vi "VDMS_FPGA_Main_8_Modules_9229.vi"() -> ()   [LabVIEW 2017]
doc: "This VI provides a template for customizing a waveform acquisition using delta-sigma based NI C Series analog input smodules."
uses:
  <vilib>/LabVIEW Targets/FPGA/cRIO/shared/nicrio_ModuleControls/nicrio_cRIO-9232_ConfigModeRing.ctl
  <vilib>/Platform/TimedLoop/XDataNode/timing_clust.ctl
  <vilib>/Platform/TimedLoop/XDataNode/nitl_modes.ctl
  <vilib>/Platform/TimedLoop/XDataNode/wakeup.ctl
  <vilib>/rvi/Emulation/niFpgaGetClockAttributes.vi
  <vilib>/rvi/Emulation/niFpgaSctlEmulationGetInTimedLoop.vi
  <vilib>/rvi/Emulation/niFpgaEmulationReportErrorSimple.vi
  <vilib>/rvi/Emulation/niFpgaProcessEmulError.vi
  <vilib>/addons/InsightCM/Devices/Shared/Cms/Fpga/AcquisitionFpgaTach/source/subVIs/Glbl Stop.vi
  <vilib>/addons/InsightCM/Devices/Shared/Cms/Fpga/AcquisitionFpgaTach/source/subVIs/FPGA Globals.vi
  <vilib>/rvi/eio/common/nirviEmuTemplateMethod_errors.vi
  <vilib>/rvi/Memory/Memory_Emulation/nirvimemoryFastEmulation.vi
  <vilib>/rvi/Memory/Memory_Emulation/nirvimemoryEmulation.vi
  <vilib>/rvi/Emulation/niFpgaEmulationIsFPGAContextNoSignature.vi
  <vilib>/rvi/DataTransferAndStorage/Container/Common/niFpgaContainerGetUniqueNameForEmu.vi
  <vilib>/rvi/errors/nirviReportUnexpectedCaseInternalError (U32).vi
  <vilib>/rvi/DataTransferAndStorage/Container/Common/niFpgaContainerExecOnDevCompGetState.vi
  <vilib>/rvi/Memory/Memory_Emulation/niFpgaMemoryEmulationCacheClearOnFirstRun.vi
  <vilib>/rvi/Memory/Memory_Emulation/nirvimemoryEmulationManagerCache_MakeExclusive.vi
  <vilib>/rvi/Memory/Memory_Emulation/niFpgaMemoryEmulationValidateCache.vi
  <vilib>/rvi/Memory/Memory_Emulation/nirvimemoryEmulationManagerCache_InsertValue.vi
  <vilib>/Utility/error.llb/Clear Errors.vi
  <vilib>/rvi/Memory/Memory_Emulation/nirvimemoryEmulationManagerCache_ReleaseExclusive.vi
  <vilib>/rvi/Memory/Memory_Emulation/nirvimemoryEmulationManagerCache_GetValue.vi
  <vilib>/rvi/Memory/Memory_Emulation/nirvimemoryEmulationManagerCache_SetValue.vi
  <vilib>/rvi/Emulation/niFpgaSctlEmulationResourceMgr.vi
  <vilib>/rvi/Emulation/niFpgaCriticalErrorInLSC.vi
  <vilib>/rvi/interface/RandomDataEmulation/niFpgaRandomDataHandleErrors.vi
  <vilib>/rvi/errors/niFpgaSetErrorForExecOnDevCompSimple.vi
  <vilib>/rvi/eio/common/nirviEmuReportErrorAndStop.vi
  <vilib>/rvi/FIFO/Fifo_Resource/nirvififoEmulationSetSize.vi
  <vilib>/rvi/FIFO/Fifo_Resource/nirviFifoEmulationQueueMgr.vi
  <instcachedir>/0/nirviFifoEmulationQueueMgr_E5CAEC123FF24DC58D834DCA3CDAA9B5.lvgen/nirviFifoEmulationQueueMgr_E5CAEC123FF24DC58D834DCA3CDAA9B5_001.vi
  <vilib>/rvi/FIFO/Fifo_Resource/nirvififoEmulationDetermineInputValidOut.vi
  <vilib>/rvi/FIFO/Fifo_Resource/nirvififoEmulationCreateLock.vi
  <vilib>/rvi/FIFO/Fifo_Resource/nirvififoEmulationObtainLock.vi
  <vilib>/rvi/FIFO/Fifo_Resource/nirvififoEmulationReleaseLock.vi
  <vilib>/rvi/occurrence/nirviWaitOnOccurrenceBase.vi
  <vilib>/rvi/errors/nirviReportUnexpectedCaseInternalError.vi
  <vilib>/eio/EIONode/EIONode.xnode
  <vilib>/rvi/DataTransferAndStorage/Container/XNode/niFpgaContainer.xnode
  <vilib>/rvi/Memory/Memory_Emulation/niFpgaMemoryEmulationRefIn.vi
  <vilib>/Platform/TimedLoop/XDataNode/XDataNode.xnode
  <vilib>/rvi/interface/RandomDataEmulation/nirviRandomDataFpgaReadWriteTemplate.vi
  <vilib>/rvi/FXPMathLib/basic elements/FxpDiscreteDelay/XNode/nifxpmath_DiscreteDelay.xnode
  <vilib>/rvi/FIFO/Fifo_Resource/niFpgaFifoEmulationRefIn.vi
  <vilib>/Platform/TimedLoop/XDataNode/XDNodeRunTimeDep.lvlib
  <vilib>/addons/InsightCM/Devices/Shared/Cms/Fpga/AcquisitionFpgaTach/source/subVIs/VibAPI_8/VDMS_VibAPI_8.lvlib
panel:
  in  "Tach Delay":u8
  out "Chassis Temperature":sgl
  in  "Enable Chan Array":bool[](array[boolean])=[FALSE, FALSE, FALSE, FALSE, FALSE, FALSE, FALSE, FALSE, FALSE, FALSE, FALSE, FALSE, FALSE, FALSE, FALSE, FALSE, FALSE, FALSE, FALSE, FALSE, FALSE, FALSE, FALSE, FALSE, FALSE, FALSE, FALSE, FALSE, FALSE, FALSE, FALSE, FALSE]
  in  "Custom Scale Intercept":sgl[](array[numeric])=[0.0, 0.0, 0.0, 0.0, 0.0, 0.0, 0.0, 0.0, 0.0, 0.0, 0.0, 0.0, 0.0, 0.0, 0.0, 0.0, 0.0, 0.0, 0.0, 0.0, 0.0, 0.0, 0.0, 0.0, 0.0, 0.0, 0.0, 0.0, 0.0, 0.0, 0.0, 0.0]
  in  "Custom Scale Slope":sgl[](array[numeric])=[0.0, 0.0, 0.0, 0.0, 0.0, 0.0, 0.0, 0.0, 0.0, 0.0, 0.0, 0.0, 0.0, 0.0, 0.0, 0.0, 0.0, 0.0, 0.0, 0.0, 0.0, 0.0, 0.0, 0.0, 0.0, 0.0, 0.0, 0.0, 0.0, 0.0, 0.0, 0.0]
  in  "Threshold2":fxp<+/-,24,7>=-10.0
  in  "Slope2":enum16{"falling", "rising"}(ring)
  in  "Hysteresis2":fxp<+/-,24,7>=1.0
  in  "Hysteresis1":fxp<+/-,24,7>=1.0
  in  "Threshold1":fxp<+/-,24,7>=-10.0
  in  "Slope1":enum16{"falling", "rising"}(ring)
  in  "Hysteresis0":fxp<+/-,24,7>=1.0
  in  "Slope0":enum16{"falling", "rising"}(ring)
  in  "Threshold0":fxp<+/-,24,7>=-10.0
  out "Tach FIFO Full":bool
  in  "Delay Comp":u32
  out "Start Trigger":bool
  in  "Number of Modules":i16=1
  out "Open Loop Chan Array":bool[](array[boolean])
  out "Short Circuit Chan Array":bool[](array[boolean])
  in  "Input Config Array":T1[](array[typedef])=[1, 1, 1, 1, 1, 1, 1, 1, 1, 1, 1, 1, 1, 1, 1, 1, 1, 1, 1, 1, 1, 1, 1, 1, 0, 0, 0, 0, 0, 0, 0, 0] items=["AC Coupled", "DC Coupled", "IEPE AC Coupled"]
  in  "Data Rate [S/s]":u32=1280
  out "Chan Count":bool
  out "Acq Loop Ticks":u32
  out "FPGA Error":errorcluster
  out "Module Underflow":bool
  out "Finished":bool
  in  "Total Avail Channels":i32=4
  in  "Samps per Chan [Finite]":i32=5120
  out "First Read":bool
  in  "Acquisition Type":enum16{"Finite Samples", "Continuous Samples"}(ring)
  out "DMA FIFO Full":bool
  in  "Stop":bool
  # "Keyphasor Info"
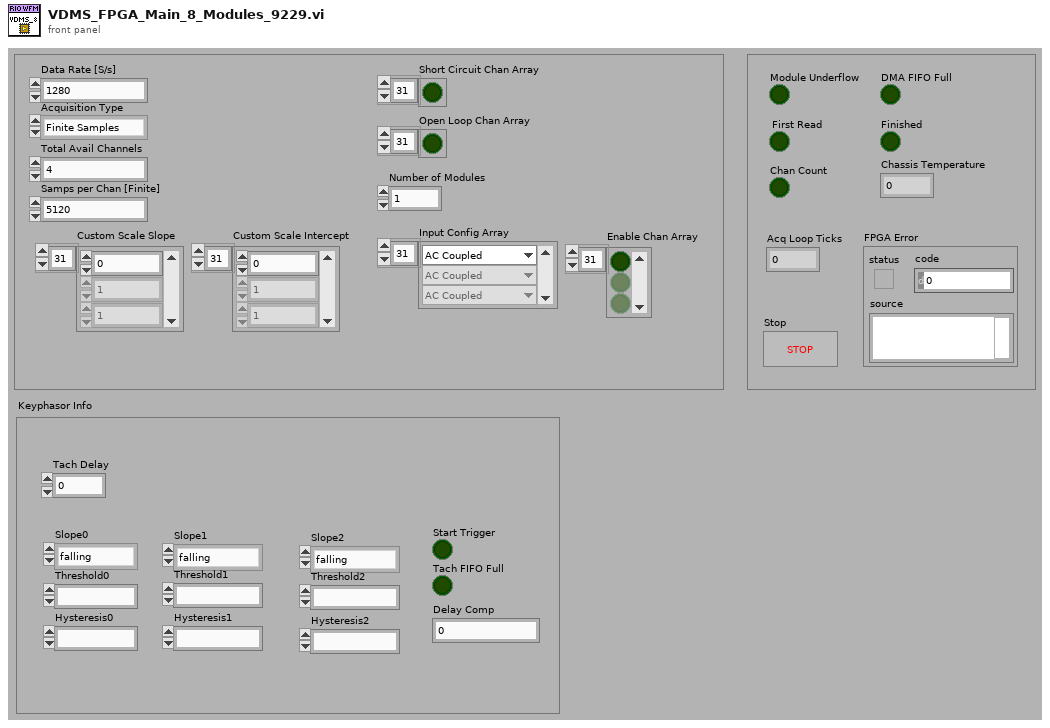
[diagram p1: front panel]
types:
  T1 = typedef "nicrio_cRIO-9232_ConfigModeRing.ctl" = u8
  T2 = typedef "XDNodeRunTimeDep.lvlib/timing_clust.ctl" = cluster{"Expected End [f-1]":u64, "Actual End [f-1]":u64, "Finished Late? [f-1]":bool, "Expected End [i-1]":u64, "Actual End [i-1]":u64, "Finished Late? [i-1]":bool, "Expected Start [i]":u64, "Actual Start [i]":u64, "Expected Start [f]":u64, "Actual Start [f]":u64, "Source Name":string, "Structure Name":string, "Period":i64, "Deadline":i64, "Offset":i64, "Start":i64, "Priority":i32, "Timeout":i32, "Mode":T3, "Wakeup Reason":T4, "Error":errorcluster, "Source Type":string, "Secondary Source Type":string, "Global End Time":u64, "Global Start Time":u64, "Frame Duration":u64, "Iteration Duration":u64, "Assigned CPU":i32, "I/O Scan Engine Mode":u32}
  T3 = typedef "XDNodeRunTimeDep.lvlib/nitl_modes.ctl" = enum32{"No Change", "Process missed periods, maintain original phase", "Discard missed periods, maintain original phase", "Process missed periods, ignore original phase", "Discard missed periods, ignore original phase"}
  T4 = typedef "XDNodeRunTimeDep.lvlib/wakeup.ctl" = enum32{"Normal", "Aborted", "Asynchronous wakeup", "Timing source error", "Timed loop error", "Timeout"}
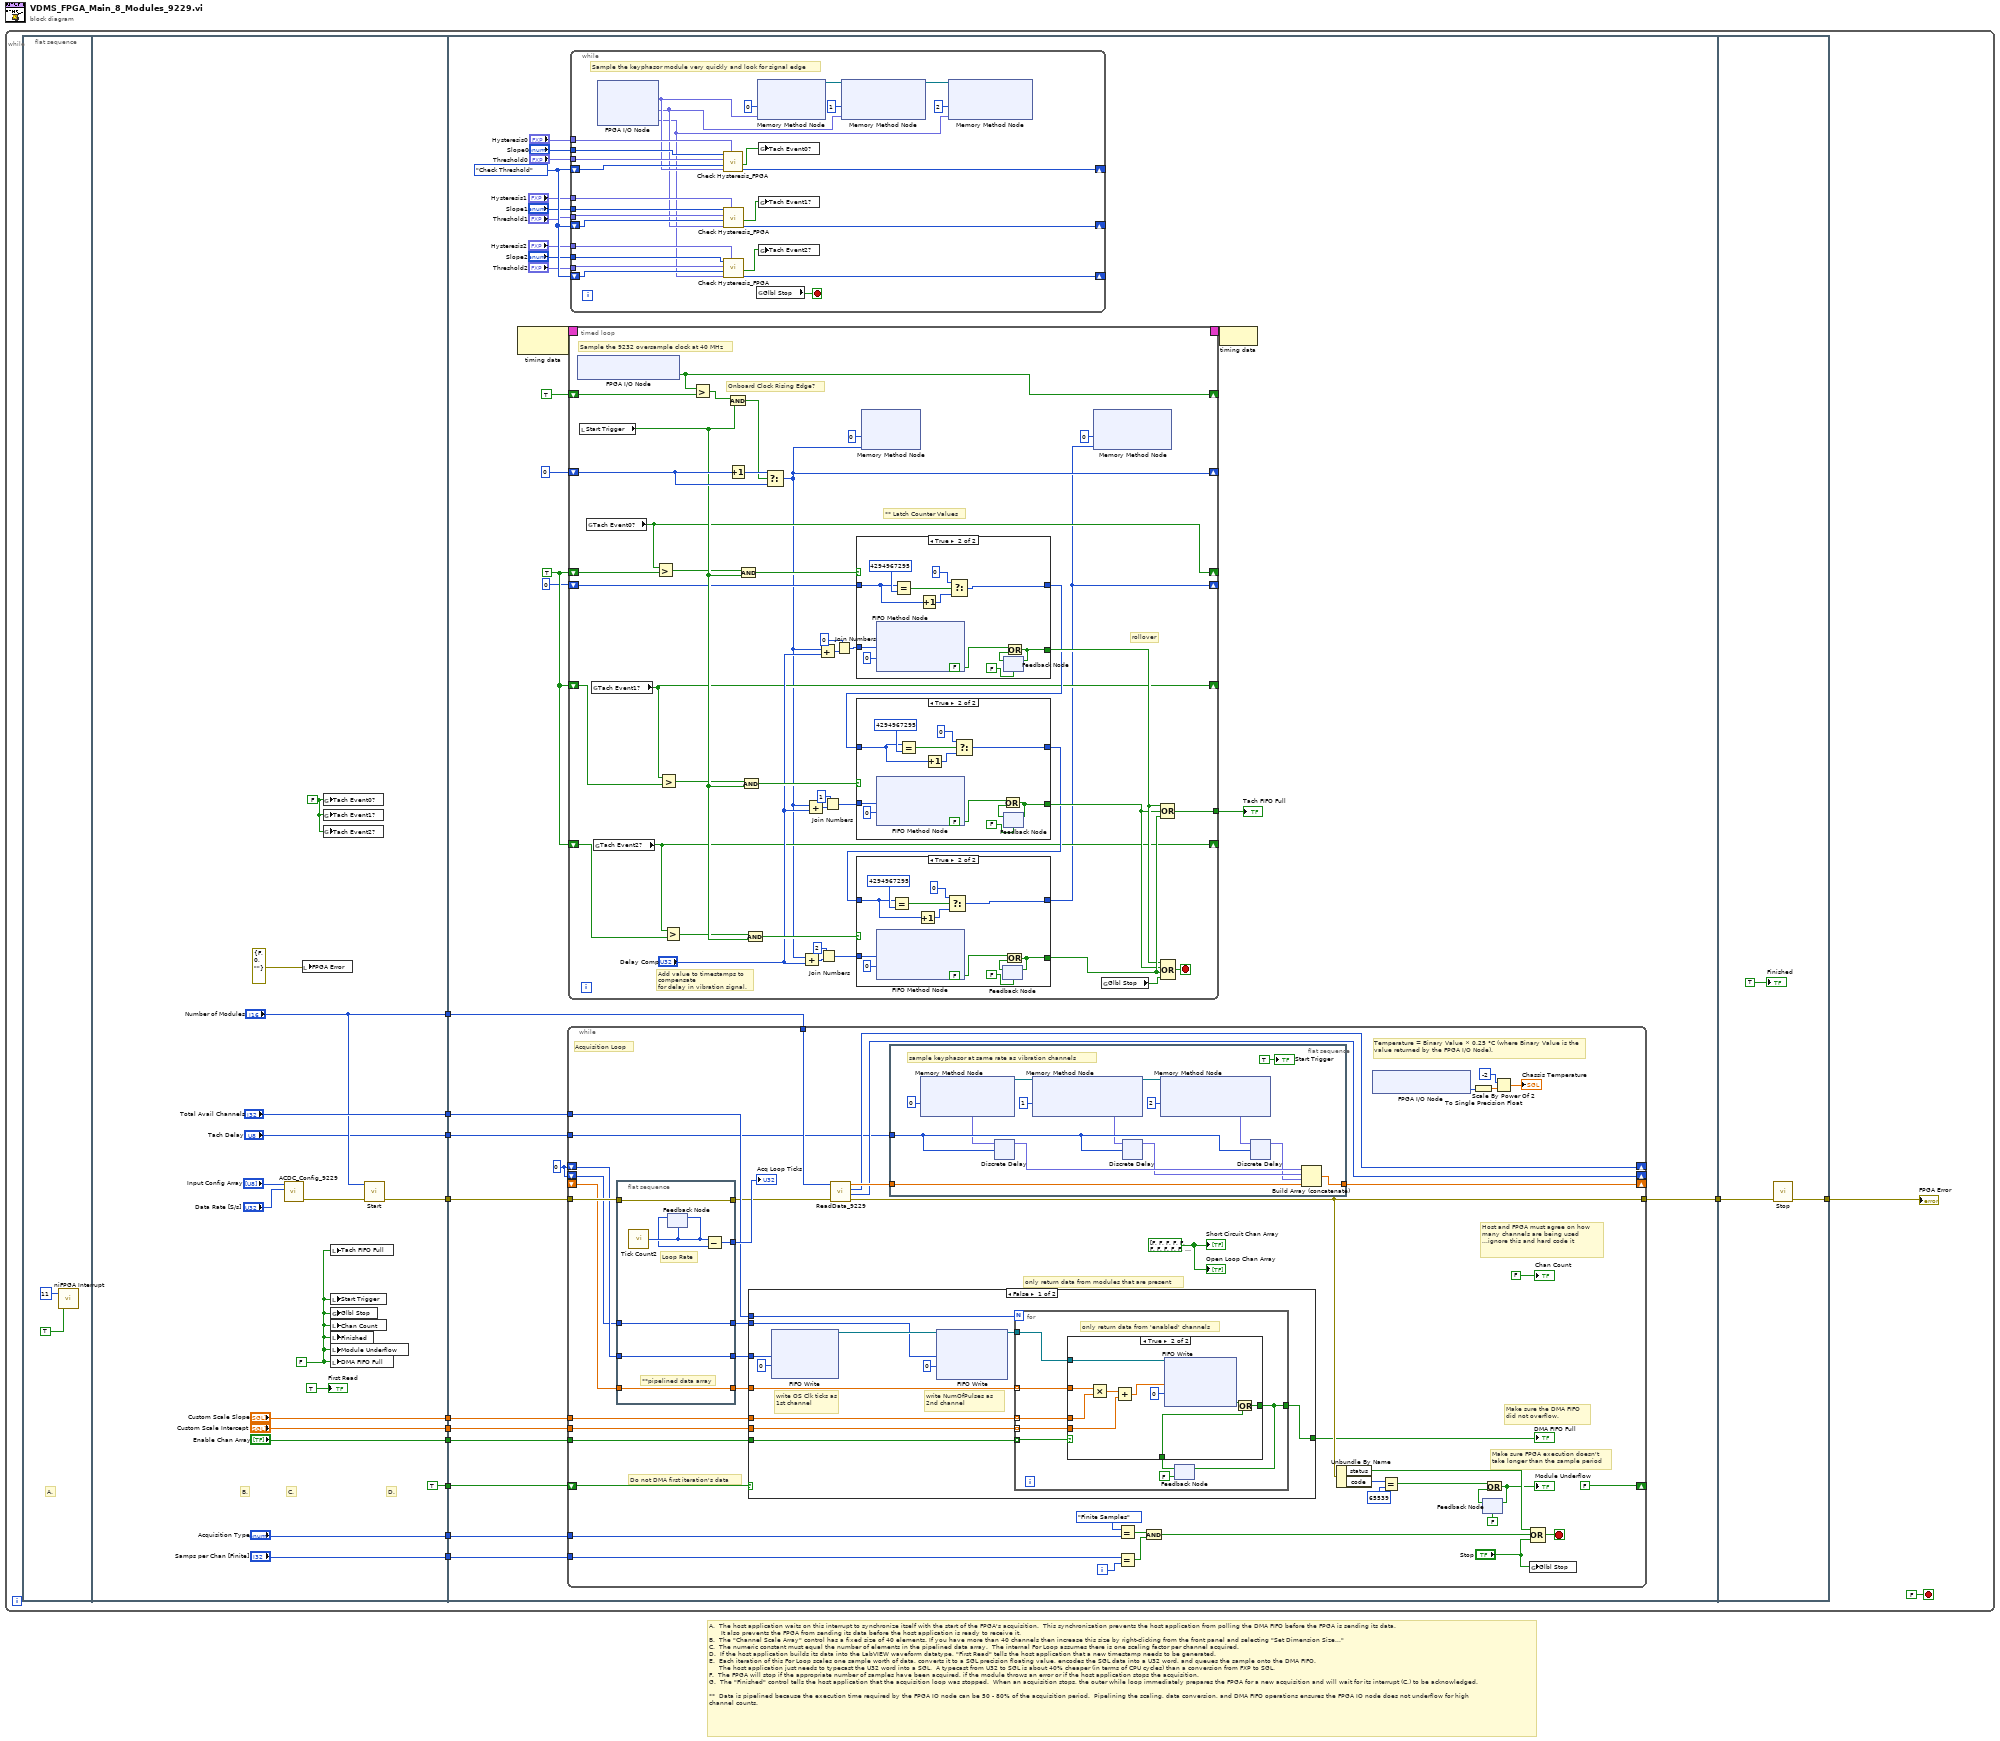
[diagram p0: block diagram]
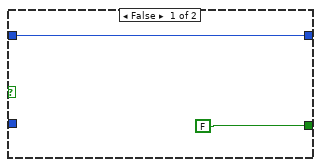
[diagram p2: hidden frame]
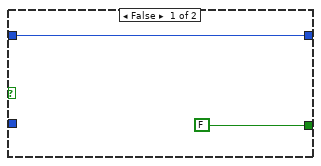
[diagram p3: hidden frame]
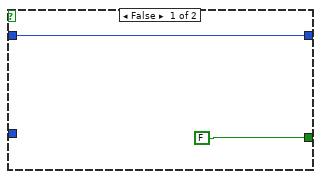
[diagram p4: hidden frame]
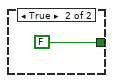
[diagram p6: hidden frame]
diagram:
  # "A.  The host application waits on this interrupt to synchronize itself with the start of the FPGA's acquisition.  This synchronization prevents the host application from polling the DMA FIFO before the FPGA is sending its data.\n      It also prevents the FPGA from sending its data before the host application is ready to receive it.\nB.  The \"Channel Scale Array\" control has a fixed size of 40 elements. If you have more than 40 channels then increase this size by right-clicking from the front panel and selecting \"Set Dimension Size...\"\nC.  The numeric constant must equal the number of elements in the pipelined data array.  The internal For Loop assumes there is one scaling factor per channel acquired.  \nD.  If the host application builds its data into the LabVIEW waveform datatype, \"First Read\" tells the host application that a new timestamp needs to be generated.\nE.  Each iteration of this For Loop scales one sample worth of data, converts it to a SGL precision floating value, encodes the SGL data into a U32 word, and queues the sample onto the DMA FIFO.  \n     The host application just needs to typecast the U32 word into a SGL.  A typecast from U32 to SGL is about 40% cheaper (in terms of CPU cycles) than a conversion from FXP to SGL.\nF.  The FPGA will stop if the appropriate number of samples have been acquired, if the module throws an error or if the host application stops the acquisition.  \nG.  The \"Finished\" control tells the host application that the acquisition loop was stopped.  When an acquisition stops, the outer while loop immediately prepares the FPGA for a new acquisition and will wait for its interrupt (C.) to be acknowledged.\n\n**  Data is pipelined because the execution time required by the FPGA IO node can be 50 - 80% of the acquisition period.  Pipelining the scaling, data conversion, and DMA FIFO operations ensures the FPGA IO node does not underflow for high\nchannel counts."
  n1 = while {
    stop <- FALSE stop-if-true
    n2 = flat-sequence {
      tunnel: [w26] -> w12
      tunnel: ["Acquisition Type"] -> w11
      tunnel: ["Samps per Chan [Finite]"] -> w10
      tunnel: ["Total Avail Channels"] -> w9
      tunnel: [TRUE ("t")] -> w8
      tunnel: ["Number of Modules"] -> w6
      tunnel: ["Custom Scale Slope"] -> w4
      tunnel: ["Custom Scale Intercept"] -> w3
      tunnel: ["Enable Chan Array"] -> w2
      tunnel: ["Tach Delay"] -> w1
      tunnel: w12 -> [w60]
      tunnel: w11 -> [w58]
      tunnel: w10 -> [w57]
      tunnel: w9 -> [w61]
      tunnel: w8 -> [w59]
      tunnel: [w56] -> w7
      tunnel: w6 -> [w55]
      tunnel: w4 -> [w38]
      tunnel: w3 -> [w37]
      tunnel: w2 -> [w36]
      tunnel: w1 -> [w33]
      tunnel: w7 -> [w277]
      tunnel: [w276] -> w5
      frame #0 {
        # "A."
        n3 = call <vilib>:"niFPGA Interrupt.vi"("Wait Until Cleared (F)"=TRUE ("Wait Until Cleared"), "IRQ Number (0)"=u8 11 ("IRQ Number")) -> ()  [unwired: 1 in]
      }
      frame #1 {
        w17 = FALSE ("Tach Event0?")
        w22 = FALSE ("Module Underflow")
        # "D."
        # "C."
        # "B."
        n4 = call <vilib>:"ACDC_Config_9229.vi"("Data Rate [S/s]"="Data Rate [S/s]", "Input Config Array"="Input Config Array") -> ("error out"=w25:errorcluster)  [unwired: 9 in]
        n5 = local write "FPGA Error"(errorcluster {"status"=FALSE, "code"=0, "source"=""} ("FPGA Error")) -> ()
        n6 = global write "FPGA Globals.vi" "Tach Event0?"(w17) -> ()
        n7 = global write "FPGA Globals.vi" "Tach Event1?"(w17) -> ()
        n8 = global write "FPGA Globals.vi" "Tach Event2?"(w17) -> ()
        n9 = local write "Tach FIFO Full"(w22) -> ()
        n10 = local write "Start Trigger"(w22) -> ()
        n11 = global write "Glbl Stop.vi" "Glbl Stop"(w22) -> ()
        n12 = local write "Chan Count"(w22) -> ()
        n13 = local write "Finished"(w22) -> ()
        n14 = local write "Module Underflow"(w22) -> ()
        n15 = local write "DMA FIFO Full"(w22) -> ()
        n16 = call <vilib>:"Start.vi"("error in (no error)"=w25, "Module Config Selector"="Number of Modules") -> ("error out"=w26:errorcluster)  [unwired: 9 in]
        "First Read" <- TRUE ("First Read")
      }
      frame #2 {
        w34 = u32 0 ("OversampleClk Ticks")
        w46 = enum16{"Check Hysteresis", "Check Threshold"}."Check Threshold" ("State Out")
        w50 = TRUE
        n17 = node-c288() -> (w54:T2)  [unwired: 1 out]
        n18 = while {
          tunnel: w60 -> [w213]
          tunnel: [w215] -> w56
          tunnel: w58 -> [w217]
          tunnel: w57 -> [w216]
          shift-right: [w192] -> _
          shift-left: _ -> [w210]
          tunnel: w61 -> [w196]
          shift-right: [FALSE ("t")] -> _
          shift-left: w59 -> [w209]
          tunnel: w55 -> [w197]
          shift-right: [w191] -> _
          shift-left: w34 -> [w190]
          tunnel: w38 -> [w188]
          tunnel: w37 -> [w187]
          tunnel: w36 -> [w186]
          shift-right: [w185] -> _
          shift-left: w34 -> [w184]
          tunnel: w33 -> [w178]
          i -> [w207]
          stop <- w220 stop-if-true
          w177 = bool[] [FALSE, FALSE, FALSE, FALSE, FALSE, FALSE, FALSE, FALSE, FALSE, FALSE, FALSE, FALSE, FALSE, FALSE, FALSE, FALSE, FALSE, FALSE, FALSE, FALSE, FALSE, FALSE, FALSE, FALSE, FALSE, FALSE, FALSE, FALSE, FALSE, FALSE, FALSE, FALSE] ("Short Circuit Chan Array")
          # "Temperature = Binary Value × 0.25 °C (where Binary Value is the value returned by the FPGA I/O Node)."
          # "only return data from modules that are present"
          # "Do not DMA first iteration's data"
          # "Acquisition Loop"
          # "Host and FPGA must agree on how \nmany channels are being used\n...ignore this and hard code it"
          # "Make sure the DMA FIFO\ndid not overflow."
          # "Make sure FPGA execution doesn't\ntake longer than the sample period"
          n19 = flat-sequence {
            tunnel: w213 -> [w271]
            tunnel: [w273] -> w212
            tunnel: w210 -> [w272]
            tunnel: [w272] -> w211
            tunnel: [w271] -> w194
            tunnel: [w270] -> w189
            tunnel: w190 -> [w270]
            tunnel: [w269] -> w183
            tunnel: w184 -> [w269]
            frame #0 {
              # "**pipelined data array"
              # "Loop Rate"
              n20 = call "Tick Count2"() -> ("Tick Count(Ticks)"=w275:u32)
              n21 = feedback-in #1(w275) -> ()
              n22 = feedback #1(w275) -> (w274:u32)
              n23 = Subtract(x=w275, y=w274) -> (x-y=w273:u32)
            }
          }
          n24 = case shown="False" w209 {
            tunnel: [w241 FALSE] -> w214
            tunnel: w211 -> [w245 _]
            tunnel: w196 -> [w246 _]
            tunnel: w189 -> [w247 _]
            tunnel: w188 -> [w244 _]
            tunnel: w187 -> [w243 _]
            tunnel: w186 -> [w242 _]
            tunnel: w183 -> [w237 _]
            frame False {
              # "write NumOfPulses as 2nd channel"
              # "write OS Clk ticks as 1st channel"
              n25 = xnode ("FIFO Write")("Element"=w247, "Timeout"=0) -> ("FIFO Out"=w240:refnum<k21>)  [unwired: 1 in, 1 out]
              n26 = xnode ("FIFO Write")("Element"=w237, "Timeout"=0, "FIFO In"=w240) -> ("FIFO Out"=w238:refnum<k21>)  [unwired: 1 out]
              n27 = for {
                N: w246 -> [_]
                tunnel: [w255] -> w241
                tunnel: w245 -> [w254] mode=indexing
                tunnel: w244 -> [w253] mode=indexing
                tunnel: w242 -> [w251] mode=indexing
                tunnel: w243 -> [w250] mode=indexing
                tunnel: w238 -> [w249]
                # "only return data from 'enabled' channels"
                n28 = feedback #2(FALSE) -> (w256:bool)
                n29 = case shown="True" w251 {
                  tunnel: w256 -> [w257 w267]
                  tunnel: [w257 w266] -> w255
                  tunnel: w254 -> [_ w265]
                  tunnel: w253 -> [_ w264]
                  tunnel: w250 -> [_ w259]
                  tunnel: w249 -> [_ w258]
                  frame False {
                  }
                  frame True {
                    n30 = Multiply(x=w265, y=w264) -> (x*y=w261:sgl)
                    n31 = Add(x=w261, y=w259) -> (x+y=w260:sgl)
                    n32 = xnode ("FIFO Write")("Element"=w260, "Timeout"=0, "FIFO In"=w258) -> ("Timed Out?"=w262:bool)  [unwired: 1 out]
                    n33 = Or(x=w262, y=w267) -> (x .or. y?=w266:bool)
                  }
                }
                n34 = feedback-in #2(w255) -> ()
              }
            }
            frame True {
            }
          }
          "DMA FIFO Full" <- w214
          n35 = call <vilib>:"ReadData_9229.vi"("error in"=w194, "Module Config Selector"=w197) -> ("error out"=w215:errorcluster, "Number Of Pulses"=w185:u32, "OversampleClk Ticks"=w191:u32, "Data Array"=w193:sgl[])  [unwired: 6 in]
          n36 = flat-sequence {
            tunnel: w193 -> [w236]
            tunnel: [w235] -> w192
            tunnel: w178 -> [w228]
            frame #0 {
              # "sample keyphasor at same rate as vibration channels"
              n37 = xnode ("Memory Method Node")("Address"=u32 0) -> ("Data"=w227:fxp<+/-,24,7>, "Memory Out"=w232:refnum<k21>)  [unwired: 1 in]
              n38 = xnode ("Discrete Delay")("D"=w227, "n-1[0..41]"=w228) -> ("Q"=w226:fxp<+/-,24,7>)
              n39 = xnode ("Memory Method Node")("Address"=u32 1, "Memory In"=w232) -> ("Data"=w225:fxp<+/-,24,7>, "Memory Out"=w231:refnum<k21>)
              n40 = xnode ("Discrete Delay")("D"=w225, "n-1[0..41]"=w228) -> ("Q"=w224:fxp<+/-,24,7>)
              n41 = xnode ("Memory Method Node")("Address"=u32 2, "Memory In"=w231) -> ("Data"=w223:fxp<+/-,24,7>)  [unwired: 1 out]
              n42 = xnode ("Discrete Delay")("D"=w223, "n-1[0..41]"=w228) -> ("Q"=w222:fxp<+/-,24,7>)
              n43 = Build Array (concatenate)(w226, w224, w222, w236) -> (w235:sgl[])
              "Start Trigger" <- TRUE ("Start Trigger")
            }
          }
          n44 = Equal?(x=enum16{"Finite Samples", "Continuous Samples"}."Finite Samples" ("y"), y=w217) -> (x = y?=w201:bool)
          n45 = Equal?(x=w216, y=w207) -> (x = y?=w200:bool)
          n46 = And(x=w201, y=w200) -> (x .and. y?=w199:bool)
          n47 = Unbundle By Name(w215) -> ("status"=w206:bool, "code"=w218:i32)
          n48 = xnode "FPGA I/O Node"() -> ("Chassis Temperature"=w180:i16)  [unwired: 1 in, 1 out]
          n49 = Equal?(x=w218, y=65539) -> (x = y?=w203:bool)
          n50 = To Single Precision Float(number=w180) -> (single precision float=w182:sgl)
          n51 = feedback #3(FALSE) -> (w205:bool)
          n52 = Or(x=w203, y=w205) -> (x .or. y?=w202:bool)
          "Module Underflow" <- w202
          n53 = feedback-in #3(w202) -> ()
          n54 = Scale By Power Of 2(n=i16 -2, x=w182) -> (x*2^n=→"Chassis Temperature":sgl)
          n55 = global write "Glbl Stop.vi" "Glbl Stop"("Stop") -> ()
          n56 = Compound Arithmetic op=OR(w206, w199, "Stop") -> (w220:bool)
          "Chan Count" <- FALSE ("Chan Count")
          "Acq Loop Ticks" <- w212
          "Short Circuit Chan Array" <- w177
          "Open Loop Chan Array" <- w177
        }
        n57 = timed-loop {
          timing: w54 -> [_]
          timing-out: [_] -> w53
          shift-right: [w92] -> _
          shift-left: u32 0 -> [w127]
          shift-right: [w129] -> _
          shift-left: TRUE -> [w130]
          shift-right: [w95] -> _
          shift-left: w50 -> [w126]
          shift-right: [w94] -> _
          shift-left: w50 -> [w120]
          shift-right: [w93] -> _
          shift-left: w50 -> [w119]
          tunnel: [w101] -> w39
          shift-right: [w91] -> _
          shift-left: u32 0 -> [w98]
          stop <- w125 stop-if-true
          # "rollover"
          # "** Latch Counter Values"
          # "Add value to timestamps to compensate \nfor delay in vibration signal."
          # "Sample the 9232 oversample clock at 40 MHz"
          # "Onboard Clock Rising Edge?"
          n58 = xnode "FPGA I/O Node"() -> ("Mod1/Onboard Clock"=w129:bool)  [unwired: 1 in, 1 out]
          n59 = local read "Start Trigger"() -> (w118:bool)
          n60 = global read "FPGA Globals.vi" "Tach Event0?"() -> (w95:bool)
          n61 = global read "FPGA Globals.vi" "Tach Event1?"() -> (w94:bool)
          n62 = global read "FPGA Globals.vi" "Tach Event2?"() -> (w93:bool)
          n63 = Greater?(x=w95, y=w126) -> (0:w117:bool)
          n64 = Greater?(x=w94, y=w120) -> (0:w116:bool)
          n65 = Greater?(x=w93, y=w119) -> (0:w115:bool)
          n66 = Greater?(x=w129, y=w130) -> (0:w124:bool)
          n67 = And(x=w124, y=w118) -> (x .and. y?=w123:bool)
          n68 = Increment(x=w127) -> (x+1=w128:u32)
          n69 = And(x=w117, y=w118) -> (x .and. y?=w114:bool)
          n70 = And(x=w116, y=w118) -> (x .and. y?=w112:bool)
          n71 = And(x=w115, y=w118) -> (x .and. y?=w106:bool)
          n72 = Select(t=w128, s=w123, f=w127) -> (s? t:f=w92:u32)
          n73 = Add(x=w92, y="Delay Comp") -> (x+y=w108:u32)
          n74 = Add(x=w92, y="Delay Comp") -> (x+y=w111:u32)
          n75 = Add(x=w92, y="Delay Comp") -> (x+y=w122:u32)
          n76 = Join Numbers(hi=u32 2, lo=w108) -> ((hi.lo)=w104:u64)
          n77 = Join Numbers(hi=u32 1, lo=w111) -> ((hi.lo)=w109:u64)
          n78 = Join Numbers(hi=u32 0, lo=w122) -> ((hi.lo)=w121:u64)
          n79 = case shown="True" w114 {
            tunnel: [FALSE w171] -> w100
            tunnel: w121 -> [_ w168]
            tunnel: w98 -> [w159 w164]
            tunnel: [w159 w161] -> w97
            frame False {
            }
            frame True {
              (unwired) FALSE
              n80 = xnode ("FIFO Method Node")("Element"=w168, "Timeout"=0) -> ("Timed Out?"=w169:bool)  [unwired: 1 in, 1 out]
              n81 = Equal?(x=w164, y=u32 4294967295) -> (x = y?=w165:bool)
              n82 = Increment(x=w164) -> (x+1=w163:u32)
              n83 = Select(t=u32 0, s=w165, f=w163) -> (s? t:f=w161:u32)
              n84 = feedback #4(FALSE) -> (w172:bool)
              n85 = Or(x=w169, y=w172) -> (x .or. y?=w171:bool)
              n86 = feedback-in #4(w171) -> ()
            }
          }
          n87 = case shown="True" w112 {
            tunnel: [FALSE w157] -> w99
            tunnel: w109 -> [_ w154]
            tunnel: w97 -> [w145 w148]
            tunnel: [w145 w147] -> w96
            frame False {
            }
            frame True {
              (unwired) FALSE
              n88 = xnode ("FIFO Method Node")("Element"=w154, "Timeout"=0) -> ("Timed Out?"=w155:bool)  [unwired: 1 in, 1 out]
              n89 = Equal?(x=w148, y=u32 4294967295) -> (x = y?=w150:bool)
              n90 = Increment(x=w148) -> (x+1=w151:u32)
              n91 = Select(t=u32 0, s=w150, f=w151) -> (s? t:f=w147:u32)
              n92 = feedback #5(FALSE) -> (w158:bool)
              n93 = Or(x=w155, y=w158) -> (x .or. y?=w157:bool)
              n94 = feedback-in #5(w157) -> ()
            }
          }
          n95 = case shown="True" w106 {
            tunnel: [FALSE w143] -> w102
            tunnel: w104 -> [_ w140]
            tunnel: w96 -> [w131 w134]
            tunnel: [w131 w133] -> w91
            frame False {
            }
            frame True {
              (unwired) FALSE
              n96 = xnode ("FIFO Method Node")("Element"=w140, "Timeout"=0) -> ("Timed Out?"=w141:bool)  [unwired: 1 in, 1 out]
              n97 = Equal?(x=w134, y=u32 4294967295) -> (x = y?=w137:bool)
              n98 = Increment(x=w134) -> (x+1=w136:u32)
              n99 = Select(t=u32 0, s=w137, f=w136) -> (s? t:f=w133:u32)
              n100 = feedback #6(FALSE) -> (w144:bool)
              n101 = Or(x=w141, y=w144) -> (x .or. y?=w143:bool)
              n102 = feedback-in #6(w143) -> ()
            }
          }
          n103 = xnode ("Memory Method Node")("Address"=u32 0, "Data"=w92) -> ()  [unwired: 1 in, 1 out]
          n104 = xnode ("Memory Method Node")("Address"=u32 0, "Data"=w91) -> ()  [unwired: 1 in, 1 out]
          n105 = global read "Glbl Stop.vi" "Glbl Stop"() -> (w103:bool)
          n106 = Compound Arithmetic op=OR(w100, w99, w102) -> (w101:bool)
          n107 = Compound Arithmetic op=OR(w100, w99, w102, w103) -> (w125:bool)
        }
        "Tach FIFO Full" <- w39
        n108 = while {
          shift-right: [w86] -> _
          shift-left: w46 -> [w87]
          tunnel: "Slope0" -> [w85]
          tunnel: "Threshold0" -> [w84]
          tunnel: "Hysteresis0" -> [w83]
          shift-right: [w82] -> _
          shift-left: w46 -> [w80]
          shift-right: [w81] -> _
          shift-left: w46 -> [w79]
          tunnel: "Hysteresis1" -> [w78]
          tunnel: "Slope1" -> [w77]
          tunnel: "Threshold1" -> [w76]
          tunnel: "Hysteresis2" -> [w75]
          tunnel: "Slope2" -> [w74]
          tunnel: "Threshold2" -> [w73]
          stop <- w88 stop-if-true
          # "Sample the keyphasor module very quickly and look for signal edge"
          n109 = xnode "FPGA I/O Node"() -> ("Mod1/AI0"=w64:fxp<+/-,24,7>, "Mod1/AI1"=w63:fxp<+/-,24,7>, "Mod1/AI2"=w62:fxp<+/-,24,7>)  [unwired: 3 in, 3 out]
          n110 = call <vilib>:"Check Hysteresis_FPGA.vi"("Hysteresis"=w83, "Analog In (Tach)"=w64, "State In"=w87, "Threshold"=w84, "Slope"=w85) -> ("State Out"=w86:enum16{"Check Hysteresis", "Check Threshold"}, "Event Ocurred?"=w71:bool)  [unwired: 2 in]
          n111 = call <vilib>:"Check Hysteresis_FPGA.vi"("Hysteresis"=w78, "Analog In (Tach)"=w63, "State In"=w80, "Threshold"=w76, "Slope"=w77) -> ("State Out"=w82:enum16{"Check Hysteresis", "Check Threshold"}, "Event Ocurred?"=w72:bool)  [unwired: 2 in]
          n112 = call <vilib>:"Check Hysteresis_FPGA.vi"("Hysteresis"=w75, "Analog In (Tach)"=w62, "State In"=w79, "Threshold"=w73, "Slope"=w74) -> ("State Out"=w81:enum16{"Check Hysteresis", "Check Threshold"}, "Event Ocurred?"=w70:bool)  [unwired: 2 in]
          n113 = global read "Glbl Stop.vi" "Glbl Stop"() -> (w88:bool)
          n114 = xnode ("Memory Method Node")("Address"=u32 0, "Data"=w64) -> ("Memory Out"=w66:refnum<k21>)  [unwired: 1 in]
          n115 = global write "FPGA Globals.vi" "Tach Event0?"(w71) -> ()
          n116 = global write "FPGA Globals.vi" "Tach Event1?"(w72) -> ()
          n117 = global write "FPGA Globals.vi" "Tach Event2?"(w70) -> ()
          n118 = xnode ("Memory Method Node")("Address"=u32 1, "Data"=w63, "Memory In"=w66) -> ("Memory Out"=w67:refnum<k21>)
          n119 = xnode ("Memory Method Node")("Address"=u32 2, "Data"=w62, "Memory In"=w67) -> ()  [unwired: 1 out]
        }
        n120 = node-c288(w53) -> ()
      }
      frame #3 {
        n121 = call <vilib>:"Stop.vi"("error in (no error)"=w277) -> ("error out"=w276:errorcluster)  [unwired: 10 in]
        "Finished" <- TRUE ("Finished")
      }
    }
    "FPGA Error" <- w5
  }
